vi "MeasAction.vi"(8 "error in (no error)":errorcluster caption="entrée d'erreur (pas d'erreur)", 9 "CurvePointIndex":i32, 10 "AllPointIndex":i32, 11 "InstrClassIn":refnum<class "SR530.lvclass"> caption="DNL_LabVIEW Object in") -> (0 "error out":errorcluster caption="sortie d'erreur", 2 "MeasDatOut":dbl[](array[numeric]), 3 "InstrClassOut":refnum<class "SR530.lvclass"> caption="DNL_LabVIEW Object out")   [LabVIEW 2019, in "SR530.lvclass"]
uses:
  SR530.lvclass
  C:/Programmes LabView/LabScanV1A/DevicesClass/BaseDevice/BaseDevice.lvclass
  SR530.lvclass/SR530.ctl
  <userlib>/SR530/Inputs.ctl
  BaseDevice/Accessor/GetClassEvent.vi
  BaseDevice/Accessor/GetClassQueue.vi
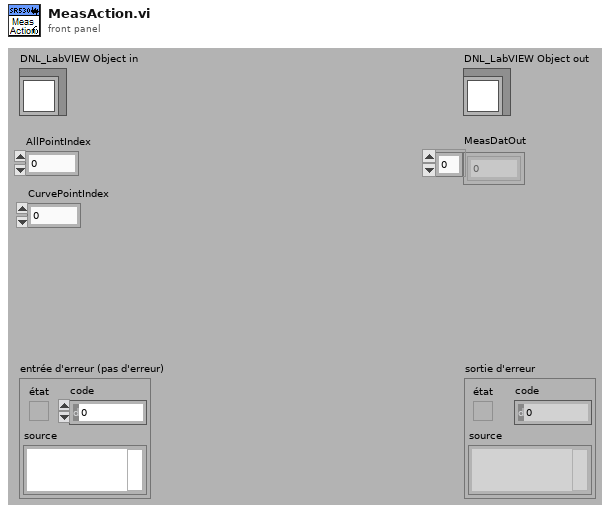
[diagram p1: front panel]
types:
  T1 = typedef "SR530.lvclass/SR530_Func.ctl" = enum16{"Read X & Y (V,V)", "Read Mag & Phase (V,°)", "Read X,Y,Mag & Phase (V,V,V,°)", "Read Analog Input (V)"}
  T2 = typedef "Inputs.ctl" = u16
  T3 = cluster{"Channel":T2, "Outputs":dbl[], "Status Byte":bool[]}
  T4 = cluster{u16, "Outputs":dbl[], "Status Byte":bool[]}
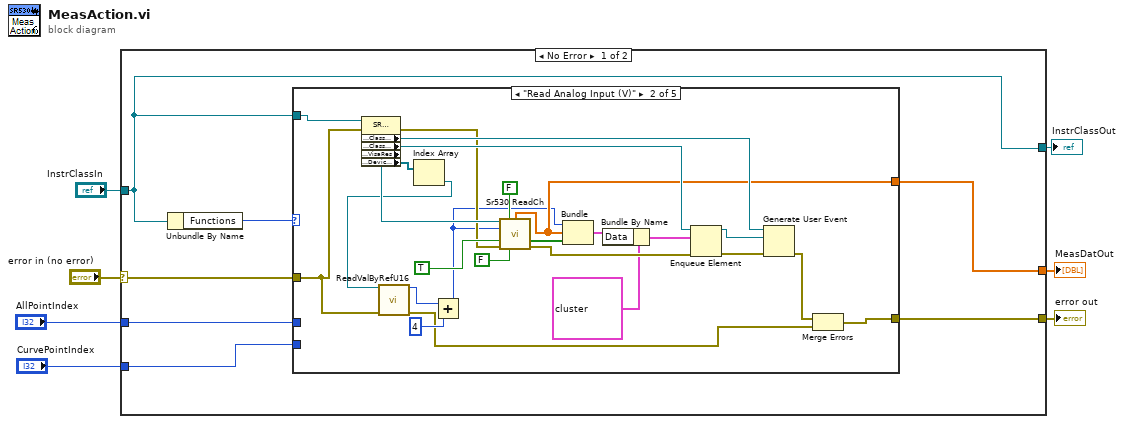
[diagram p0: block diagram]
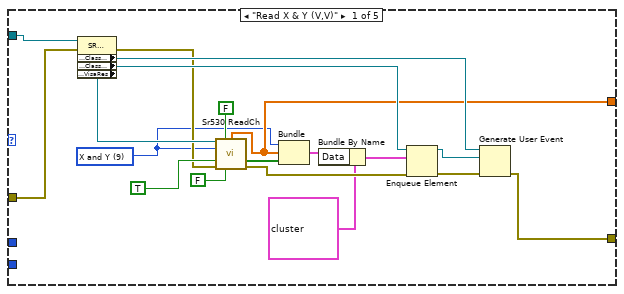
[diagram p2: hidden frame]
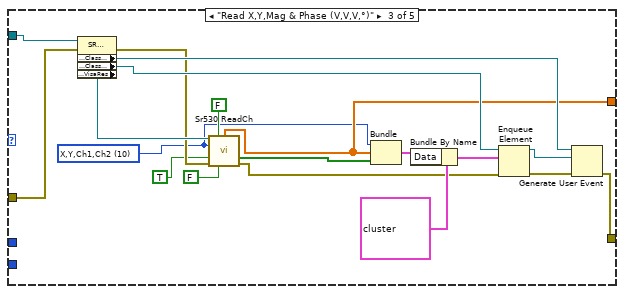
[diagram p3: hidden frame]
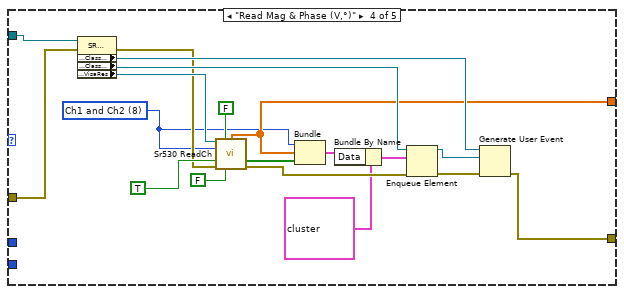
[diagram p4: hidden frame]
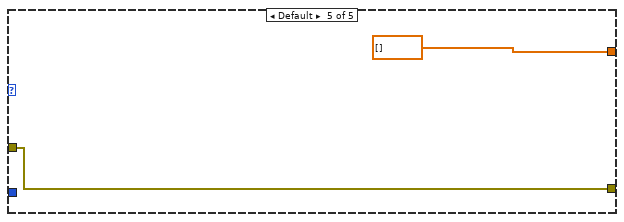
[diagram p5: hidden frame]
diagram:
  n1 = case shown="No Error" "error in (no error)" {
    selector: "error in (no error)" -> [w10 w99]
    tunnel: "InstrClassIn" -> [w8 w100]
    tunnel: [w8 w100] -> w5
    tunnel: "AllPointIndex" -> [w14 _]
    tunnel: [w13 w99] -> w3
    tunnel: [w12 _] -> w2
    tunnel: "CurvePointIndex" -> [w9 _]
    frame No Error {
      n2 = Unbundle By Name(w8) -> ("Functions"=w11:T1)
      n3 = case shown="\"Read Analog Input (V)\"" w11 {
        tunnel: w14 -> [_ _ _ _ _]
        tunnel: [w17 w35 w65 w80 w98] -> w13
        tunnel: [w16 w42 w60 w79 dbl[] [] ("Outputs")] -> w12
        tunnel: w10 -> [w18 w36 w66 w81 w98]
        tunnel: w9 -> [_ _ _ _ _]
        tunnel: w8 -> [w19 w44 w67 w82 _]
        frame "Read X & Y (V,V)" {
          w15 = T2 9 items=["Channel 1", "X Output", "Channel 2", "Y Output", "X1", "X2", "X3", "X4", "Ch1 and Ch2", "X and Y", "X,Y,Ch1,Ch2"] ("Channel")
          n4 = property class="SR530.lvclass"(reference=w19, error in=w18) -> (error out=w20:errorcluster, "Accessor:ClassEvent"=w30:refnum<user-event>, "Accessor:ClassQueue"=w24:refnum<queue>, "Accessor:VisaRes"=w33:refnum<visa-resource-name>)  [unwired: 1 out]
          n5 = call <userlib>:"Sr530 ReadCh.vi"("VISA Rsrc"=w33, "Autoscale"=FALSE, "Channel"=w15, "Check Status"=TRUE, "error in (no error)"=w20, "Ask Correction"=FALSE) -> ("Outputs"=w16:dbl[], "Status Byte"=w27:bool[], "error out"=w29:errorcluster)  [unwired: 2 in, 5 out]
          n6 = Bundle("Channel"=w15, "Outputs"=w16, "Status Byte"=w27) -> (w28:T3)  [unwired: 1 in]
          n7 = Bundle By Name(cluster=cluster{"Message":string, "Data":variant, i32} {"Message"="MeasDone", "Data"=variant, 0} ("élément"), "Data"=w28) -> (w26:cluster{"Message":string, "Data":variant, i32})
          n8 = Enqueue Element(queue=w24, element=w26, error in (no error)=w29) -> (queue out=w32:refnum<queue>, error out=w31:errorcluster)  [unwired: 1 in, 1 out]
          n9 = Generate User Event(user event=w30, event data cluster=w32, error in=w31) -> (error out=w17:errorcluster)  [unwired: 1 in, 1 out]
        }
        frame "Read Analog Input (V)" {
          n10 = property class="SR530.lvclass"(reference=w44, error in=w36) -> (error out=w45:errorcluster, "Accessor:ClassEvent"=w55:refnum<user-event>, "Accessor:ClassQueue"=w49:refnum<queue>, "Accessor:VisaRes"=w58:refnum<visa-resource-name>, "Accessor:DeviceCtrl"=w41:refnum<vi>[])  [unwired: 1 out]
          n11 = Index Array(array=w41) -> (element=w40:refnum<vi>)  [unwired: 1 in]
          n12 = call <userlib>:"ReadValByRefU16.vi"("Control Ref"=w40, "error in"=w36) -> ("Valeur"=w39:u16, "error out"=w34:errorcluster)  [unwired: 12 in]
          n13 = Add(x=w39, y=u16 4) -> (x+y=w37:u16)
          n14 = call <userlib>:"Sr530 ReadCh.vi"("VISA Rsrc"=w58, "Autoscale"=FALSE, "Channel"=w37, "Check Status"=TRUE, "error in (no error)"=w45, "Ask Correction"=FALSE) -> ("Outputs"=w42:dbl[], "Status Byte"=w52:bool[], "error out"=w54:errorcluster)  [unwired: 2 in, 5 out]
          n15 = Bundle(w37, "Outputs"=w42, "Status Byte"=w52) -> (w53:T4)  [unwired: 1 in]
          n16 = Bundle By Name(cluster=cluster{"Message":string, "Data":variant, i32} {"Message"="MeasDone", "Data"=variant, 0} ("élément"), "Data"=w53) -> (w51:cluster{"Message":string, "Data":variant, i32})
          n17 = Enqueue Element(queue=w49, element=w51, error in (no error)=w54) -> (queue out=w57:refnum<queue>, error out=w56:errorcluster)  [unwired: 1 in, 1 out]
          n18 = Generate User Event(user event=w55, event data cluster=w57, error in=w56) -> (error out=w43:errorcluster)  [unwired: 1 in, 1 out]
          n19 = Merge Errors(w43, w34) -> (w35:errorcluster)
        }
        frame "Read X,Y,Mag & Phase (V,V,V,°)" {
          w59 = T2 10 items=["Channel 1", "X Output", "Channel 2", "Y Output", "X1", "X2", "X3", "X4", "Ch1 and Ch2", "X and Y", "X,Y,Ch1,Ch2"] ("Channel")
          n20 = property class="SR530.lvclass"(reference=w67, error in=w66) -> (error out=w68:errorcluster, "Accessor:ClassEvent"=w74:refnum<user-event>, "Accessor:ClassQueue"=w69:refnum<queue>, "Accessor:VisaRes"=w77:refnum<visa-resource-name>)  [unwired: 1 out]
          n21 = call <userlib>:"Sr530 ReadCh.vi"("VISA Rsrc"=w77, "Autoscale"=FALSE, "Channel"=w59, "Check Status"=TRUE, "error in (no error)"=w68, "Ask Correction"=FALSE) -> ("Outputs"=w60:dbl[], "Status Byte"=w72:bool[], "error out"=w61:errorcluster)  [unwired: 2 in, 5 out]
          n22 = Bundle("Channel"=w59, "Outputs"=w60, "Status Byte"=w72) -> (w73:T3)  [unwired: 1 in]
          n23 = Bundle By Name(cluster=cluster{"Message":string, "Data":variant, i32} {"Message"="MeasDone", "Data"=variant, 0} ("élément"), "Data"=w73) -> (w71:cluster{"Message":string, "Data":variant, i32})
          n24 = Enqueue Element(queue=w69, element=w71, error in (no error)=w61) -> (queue out=w76:refnum<queue>, error out=w75:errorcluster)  [unwired: 1 in, 1 out]
          n25 = Generate User Event(user event=w74, event data cluster=w76, error in=w75) -> (error out=w65:errorcluster)  [unwired: 1 in, 1 out]
        }
        frame "Read Mag & Phase (V,°)" {
          w78 = T2 8 items=["Channel 1", "X Output", "Channel 2", "Y Output", "X1", "X2", "X3", "X4", "Ch1 and Ch2", "X and Y", "X,Y,Ch1,Ch2"] ("Channel")
          n26 = property class="SR530.lvclass"(reference=w82, error in=w81) -> (error out=w83:errorcluster, "Accessor:ClassEvent"=w93:refnum<user-event>, "Accessor:ClassQueue"=w87:refnum<queue>, "Accessor:VisaRes"=w96:refnum<visa-resource-name>)  [unwired: 1 out]
          n27 = call <userlib>:"Sr530 ReadCh.vi"("VISA Rsrc"=w96, "Autoscale"=FALSE, "Channel"=w78, "Check Status"=TRUE, "error in (no error)"=w83, "Ask Correction"=FALSE) -> ("Outputs"=w79:dbl[], "Status Byte"=w90:bool[], "error out"=w92:errorcluster)  [unwired: 2 in, 5 out]
          n28 = Bundle("Channel"=w78, "Outputs"=w79, "Status Byte"=w90) -> (w91:T3)  [unwired: 1 in]
          n29 = Bundle By Name(cluster=cluster{"Message":string, "Data":variant, i32} {"Message"="MeasDone", "Data"=variant, 0} ("élément"), "Data"=w91) -> (w89:cluster{"Message":string, "Data":variant, i32})
          n30 = Enqueue Element(queue=w87, element=w89, error in (no error)=w92) -> (queue out=w95:refnum<queue>, error out=w94:errorcluster)  [unwired: 1 in, 1 out]
          n31 = Generate User Event(user event=w93, event data cluster=w95, error in=w94) -> (error out=w80:errorcluster)  [unwired: 1 in, 1 out]
        }
        frame Default {
        }
      }
    }
    frame Error {
    }
  }
  "error out" <- w3
  "InstrClassOut" <- w5
  "MeasDatOut" <- w2
